vi "delete me.vi"() -> ()   [LabVIEW 2020]
uses:
  Shared/GUI_Template/GUI_master/tcp_new_data_event.ctl
  Shared/GUI_Template/GUI_master/tcp new data cluster.ctl
  <vilib>/Utility/file.llb/Read From Spreadsheet File (string).vi
panel:
  out "millisecond timer value":u32
  out "appended path":path
  in  "GUIdevice 98":string="PicoPad4"
  in  "Position.Axis 111::98":dbl=77.0 caption="Motor Axis 1" min=-30000.0 max=30000.0 format="%#_6f"
  in  "Position.Axis 112::98":dbl=77.0 caption="Motor Axis 1" min=-20000.0 max=20000.0 format="%#_6f"
  in  "Position.Axis 113::98":dbl=77.0 caption="Motor Axis 1" min=-20000.0 max=20000.0 format="%#_6f"
  in  "Position.Axis 121::98":dbl=77.0 caption="Motor Axis 1" min=-999999.0 max=999999.0 format="%#_6f"
  in  "Position.Axis 122::98":dbl=77.0 caption="Motor Axis 1" min=-999999.0 max=999999.0 format="%#_6f"
  in  "Position.Axis 123::98":dbl=77.0 caption="Motor Axis 1" min=-999999.0 max=999999.0 format="%#_6f"
  in  "Position.Axis 131::98":dbl=77.0 caption="Motor Axis 1" min=-999999.0 max=999999.0 format="%#_6f"
  in  "Position.Axis 132::98":dbl=77.0 caption="Motor Axis 1" min=-999999.0 max=999999.0 format="%#_6f"
  in  "Position.Axis 133::98":dbl=77.0 caption="Motor Axis 1" min=-999999.0 max=999999.0 format="%#_6f"
  in  "Position.Axis 141::98":dbl=77.0 caption="Motor Axis 1" min=-999999.0 max=999999.0 format="%#_6f"
  in  "Position.Axis 142::98":dbl=77.0 caption="Motor Axis 1" min=-999999.0 max=999999.0 format="%#_6f"
  in  "Position.Axis 143::98":dbl=77.0 caption="Motor Axis 1" min=-999999.0 max=999999.0 format="%#_6f"
  in  "Position.Axis 211::98":dbl=77.0 caption="Motor Axis 1" min=-999999.0 max=999999.0 format="%#_6f"
  in  "Position.Axis 212::98":dbl=77.0 caption="Motor Axis 1" min=-999999.0 max=999999.0 format="%#_6f"
  in  "Position.Axis 213::98":dbl=77.0 caption="Motor Axis 1" min=-999999.0 max=999999.0 format="%#_6f"
  in  "Position.Axis 221::98":dbl=77.0 caption="Motor Axis 1" min=-999999.0 max=999999.0 format="%#_6f"
  in  "Position.Axis 222::98":dbl=77.0 caption="Motor Axis 1" min=-999999.0 max=999999.0 format="%#_6f"
  in  "Position.Axis 223::98":dbl=77.0 caption="Motor Axis 1" min=-999999.0 max=999999.0 format="%#_6f"
  in  "Position.Axis 231::98":dbl=77.0 caption="Motor Axis 1" min=-999999.0 max=999999.0 format="%#_6f"
  in  "Position.Axis 232::98":dbl=77.0 caption="Motor Axis 1" min=-999999.0 max=999999.0 format="%#_6f"
  in  "Position.Axis 233::98":dbl=77.0 caption="Motor Axis 1" min=-999999.0 max=999999.0 format="%#_6f"
  in  "Position.Axis 241::98":dbl=77.0 caption="Motor Axis 1" min=-999999.0 max=999999.0 format="%#_6f"
  in  "Position.Axis 242::98":dbl=77.0 caption="Motor Axis 1" min=-999999.0 max=999999.0 format="%#_6f"
  in  "Position.Axis 243::98":dbl=77.0 caption="Motor Axis 1" min=-999999.0 max=999999.0 format="%#_6f"
  in  "Position.Axis 311::98":dbl=77.0 caption="Motor Axis 1" min=-999999.0 max=999999.0 format="%#_6f"
  in  "Position.Axis 312::98":dbl=77.0 caption="Motor Axis 1" min=-999999.0 max=999999.0 format="%#_6f"
  in  "Position.Axis 313::98":dbl=77.0 caption="Motor Axis 1" min=-999999.0 max=999999.0 format="%#_6f"
  in  "Position.Axis 321::98":dbl=77.0 caption="Motor Axis 1" min=-999999.0 max=999999.0 format="%#_6f"
  in  "Position.Axis 322::98":dbl=77.0 caption="Motor Axis 1" min=-999999.0 max=999999.0 format="%#_6f"
  in  "Position.Axis 323::98":dbl=77.0 caption="Motor Axis 1" min=-999999.0 max=999999.0 format="%#_6f"
  in  "Position.Axis 331::98":dbl=77.0 caption="Motor Axis 1" min=-999999.0 max=999999.0 format="%#_6f"
  in  "Position.Axis 332::98":dbl=77.0 caption="Motor Axis 1" min=-999999.0 max=999999.0 format="%#_6f"
  in  "Position.Axis 333::98":dbl=77.0 caption="Motor Axis 1" min=-999999.0 max=999999.0 format="%#_6f"
  in  "Position.Axis 341::98":dbl=77.0 caption="Motor Axis 1" min=-999999.0 max=999999.0 format="%#_6f"
  in  "Position.Axis 342::98":dbl=77.0 caption="Motor Axis 1" min=-999999.0 max=999999.0 format="%#_6f"
  in  "Position.Axis 343::98":dbl=77.0 caption="Motor Axis 1" min=-999999.0 max=999999.0 format="%#_6f"
  in  "Position.Axis 411::98":dbl=77.0 caption="Motor Axis 1" min=-999999.0 max=999999.0 format="%#_6f"
  in  "Position.Axis 412::98":dbl=77.0 caption="Motor Axis 1" min=-999999.0 max=999999.0 format="%#_6f"
  in  "Position.Axis 413::98":dbl=77.0 caption="Motor Axis 1" min=-999999.0 max=999999.0 format="%#_6f"
  in  "Position.Axis 421::98":dbl=77.0 caption="Motor Axis 1" min=-999999.0 max=999999.0 format="%#_6f"
  in  "Position.Axis 422::98":dbl=77.0 caption="Motor Axis 1" min=-999999.0 max=999999.0 format="%#_6f"
  in  "Position.Axis 423::98":dbl=77.0 caption="Motor Axis 1" min=-999999.0 max=999999.0 format="%#_6f"
  in  "Position.Axis 431::98":dbl=77.0 caption="Motor Axis 1" min=-999999.0 max=999999.0 format="%#_6f"
  in  "Position.Axis 432::98":dbl=77.0 caption="Motor Axis 1" min=-999999.0 max=999999.0 format="%#_6f"
  in  "Position.Axis 433::98":dbl=77.0 caption="Motor Axis 1" min=-999999.0 max=999999.0 format="%#_6f"
  in  "Position.Axis 441::98":dbl=77.0 caption="Motor Axis 1" min=-999999.0 max=999999.0 format="%#_6f"
  in  "Position.Axis 442::98":dbl=77.0 caption="Motor Axis 1" min=-999999.0 max=999999.0 format="%#_6f"
  in  "Position.Axis 443::98":dbl=77.0 caption="Motor Axis 1" min=-999999.0 max=999999.0 format="%#_6f"
  in  "Position.Axis 511::98":dbl=77.0 caption="Motor Axis 1" min=-999999.0 max=999999.0 format="%#_6f"
  in  "Position.Axis 512::98":dbl=77.0 caption="Motor Axis 1" min=-999999.0 max=999999.0 format="%#_6f"
  in  "Position.Axis 513::98":dbl=77.0 caption="Motor Axis 1" min=-999999.0 max=999999.0 format="%#_6f"
  in  "Position.Axis 521::98":dbl=77.0 caption="Motor Axis 1" min=-999999.0 max=999999.0 format="%#_6f"
  in  "Position.Axis 522::98":dbl=77.0 caption="Motor Axis 1" min=-999999.0 max=999999.0 format="%#_6f"
  in  "Position.Axis 523::98":dbl=77.0 caption="Motor Axis 1" min=-999999.0 max=999999.0 format="%#_6f"
  in  "Position.Axis 531::98":dbl=77.0 caption="Motor Axis 1" min=-999999.0 max=999999.0 format="%#_6f"
  in  "Position.Axis 532::98":dbl=77.0 caption="Motor Axis 1" min=-999999.0 max=999999.0 format="%#_6f"
  in  "Position.Axis 533::98":dbl=77.0 caption="Motor Axis 1" min=-999999.0 max=999999.0 format="%#_6f"
  in  "Position.Axis 541::98":dbl=77.0 caption="Motor Axis 1" min=-999999.0 max=999999.0 format="%#_6f"
  in  "Position.Axis 542::98":dbl=77.0 caption="Motor Axis 1" min=-999999.0 max=999999.0 format="%#_6f"
  in  "Position.Axis 543::98":dbl=77.0 caption="Motor Axis 1" min=-999999.0 max=999999.0 format="%#_6f"
  in  "Numeric":dbl
  out "CCDs":string[](array[string])
  in  "GUIdevice 12":string
  in  "GUIdevice 11":string
  in  "GUIdevice 10":string
  in  "GUIdevice 9":string
  out "error out 2":errorcluster
  out "Names":string[](array[string])
  in  "Tab Control 2":enum32{"Config ", "Main", "History"}(tab)=enum."Main"
  out "Cameras":T1
  in  "Exposure:12":dbl=0.095 min=0.0001 max=1.0 format="%#_6f"
  in  "Triggerdelay::12":dbl=0.003 min=0.0 max=0.09 format="%#_6f"
  in  "Exposure::11":dbl=0.095 min=0.0001 max=1.0 format="%#_6f"
  in  "Triggerdelay::11":dbl=0.003 min=0.0 max=0.09 format="%#_6f"
  in  "Exposure::10":dbl=0.095 min=0.0001 max=1.0 format="%#_6f"
  in  "Triggerdelay::10":dbl=0.003 min=0.0 max=0.09 format="%#_6f"
  in  "Exposure::9":dbl=0.095 min=0.0001 max=1.0 format="%#_6f"
  in  "Triggerdelay::9":dbl=0.003 min=0.0 max=0.09 format="%#_6f"
  in  "Trigger::9":bool
  in  "Trigger::10":bool caption="Trigger:10"
  in  "Trigger::11":bool
  in  "Trigger::12":bool
  in  "Exposure::8":dbl=0.095 caption="sdgdfg" min=0.0001 max=1.0 format="%#_6f"
  in  "Triggerdelay::8":dbl=0.003 caption="sdfsd" min=0.0 max=0.09 format="%#_6f"
  in  "Trigger::8":bool
  in  "Exposure::7":dbl=0.095 caption="dfgdf" min=0.0001 max=1.0 format="%#_6f"
  in  "Triggerdelay::7":dbl=0.003 caption="dfgdfg" min=0.0 max=0.09 format="%#_6f"
  in  "Trigger::7":bool
  in  "Exposure::6":dbl=0.095 caption="dfgdfg" min=0.0001 max=1.0 format="%#_6f"
  in  "Triggerdelay::6":dbl=0.003 caption="dfgdfg" min=0.0 max=0.09 format="%#_6f"
  in  "Trigger::6":bool
  in  "Exposure::5":dbl=0.095 caption="dfgfd" min=1e-05 max=2.0 format="%#_6f"
  in  "Triggerdelay::5":dbl=0.003 caption="dfgdf" min=0.0 max=100000.0 format="%#_6f"
  in  "Trigger::5":bool
  in  "Exposure::4":dbl=0.095 caption="dfgdf" min=0.0001 max=1.0 format="%#_6f"
  in  "Triggerdelay::4":dbl=0.003 caption="dfgdfgfd" min=0.0 max=0.09 format="%#_6f"
  in  "Trigger::4":bool
  in  "Exposure::3":dbl=0.095 caption="dfgdf" min=1e-05 max=2.0 format="%#_6f"
  in  "Triggerdelay::3":dbl=0.003 caption="dfgdfg" min=0.0 max=0.09 format="%#_6f"
  in  "Trigger::3":bool
  in  "Exposure::2":dbl=0.095 caption="gfdg" min=0.0001 max=1.0 format="%#_6f"
  in  "Triggerdelay::2":dbl=0.003 caption="dfgdfg" min=0.0 max=0.09 format="%#_6f"
  in  "Trigger::2":bool
  out "image::1":T2(plugin-control) caption="regen-out-cam"
  out "image::2":T2(plugin-control) caption="xpw-cam"
  out "image::3":T2(plugin-control) caption="xpw-out-cam"
  out "image::4":T2(plugin-control) caption="amp0-out-cam"
  out "image::5":T2(plugin-control) caption="preamp-in-cam"
  out "image::6":T2(plugin-control) caption="preamp-2nd-pass-cam"
  out "image::7":T2(plugin-control) caption="compressor-in-cam"
  out "image::8":T2(plugin-control) caption="compressor-out-cam"
  in  "Exposure::1":dbl=0.095 caption="exposure" min=0.0001 max=1.0 format="%#_6f"
  in  "Triggerdelay::1":dbl=0.003 caption="trig delay" min=0.0 max=0.09 format="%#_6f"
  in  "Trigger::1":bool
  in  "UDP error message":string
  out "image::9":T2(plugin-control)
  out "image::10":T2(plugin-control)
  out "image::11":T2(plugin-control)
  out "image::12":T2(plugin-control)
  in  "Feedback Global":bool
  in  "GUIdevice 8":string="B5_CompressorOut"
  in  "Tab Control":T3(tab)
  in  "Center":bool
  in  "Save Stats":bool
  in  "Save Config":bool
  in  "Load Config":bool
  in  "Img to avg":i32=3 min=3 max=200
  in  "Reset History":bool
  in  "new tdms":bool
  in  "deivice ini":bool
  in  "RelativeMove.Axis 1.CCW::99":bool caption="RelativeMove.Axis 1.CCW::1"
  in  "RelativeMove.Axis 1.CW::99":bool caption="RelativeMove.Axis 1.CW::1"
  in  "RelativeMove.Axis 2.CCW::99":bool caption="RelativeMove.Axis. 2.CCW::1"
  in  "RelativeMove.Axis 2.CW::99":bool caption="RelativeMove.Axis 2.CW::1"
  in  "RelativeSettings.Axis 1.Position::99":dbl caption="Axis 1 Position" min=-999999.0 max=999999.0 format="%_4p"
  in  "RelativeSettings.Axis 2.Position::99":dbl caption="Axis 2 Position" min=-999999.0 max=999999.0 format="%_4p"
  in  "RelativeSettings.Axis 2.StepSize::99":dbl=50.0 caption="Axis 2 StepSize" min=0.0 max=999999.0 format="%_4p"
  in  "RelativeSettings.Axis 1.StepSize::99":dbl=50.0 caption="Axis 1 Stepsize" min=0.0 max=999999.0 format="%_4p"
  in  "CCDs":u16(ring) items=["regen-out-cam", "xpw-cam", "xpw-out-cam", "amp0-out-cam", "preamp-in-cam", "preamp-2nd-pass-cam", "compressor-in-cam", "compressor-out-cam", "", "", "", ""]
  out "motor refs":refnum<vi>[](array[refnum])
  in  "Position.Axis 511::99":dbl=77.0 caption="Motor Axis 1" min=-999999.0 max=999999.0 format="%#_6f"
  in  "Position.Axis 512::99":dbl=77.0 caption="Motor Axis 1" min=-999999.0 max=999999.0 format="%#_6f"
  in  "Position.Axis 513::99":dbl=77.0 caption="Motor Axis 1" min=-999999.0 max=999999.0 format="%#_6f"
  in  "Position.Axis 521::99":dbl=77.0 caption="Motor Axis 1" min=-999999.0 max=999999.0 format="%#_6f"
  in  "Position.Axis 522::99":dbl=77.0 caption="Motor Axis 1" min=-999999.0 max=999999.0 format="%#_6f"
  in  "Position.Axis 523::99":dbl=77.0 caption="Motor Axis 1" min=-999999.0 max=999999.0 format="%#_6f"
  in  "Position.Axis 531::99":dbl=77.0 caption="Motor Axis 1" min=-999999.0 max=999999.0 format="%#_6f"
  in  "Position.Axis 532::99":dbl=77.0 caption="Motor Axis 1" min=-999999.0 max=999999.0 format="%#_6f"
  in  "Position.Axis 533::99":dbl=77.0 caption="Motor Axis 1" min=-999999.0 max=999999.0 format="%#_6f"
  in  "Position.Axis 541::99":dbl=77.0 caption="Motor Axis 1" min=-999999.0 max=999999.0 format="%#_6f"
  in  "Position.Axis 542::99":dbl=77.0 caption="Motor Axis 1" min=-999999.0 max=999999.0 format="%#_6f"
  in  "Position.Axis 543::99":dbl=77.0 caption="Motor Axis 1" min=-999999.0 max=999999.0 format="%#_6f"
  in  "Position.Axis 411::99":dbl=77.0 caption="Motor Axis 1" min=-999999.0 max=999999.0 format="%#_6f"
  in  "Position.Axis 412::99":dbl=77.0 caption="Motor Axis 1" min=-999999.0 max=999999.0 format="%#_6f"
  in  "Position.Axis 413::99":dbl=77.0 caption="Motor Axis 1" min=-999999.0 max=999999.0 format="%#_6f"
  in  "Position.Axis 421::99":dbl=77.0 caption="Motor Axis 1" min=-999999.0 max=999999.0 format="%#_6f"
  in  "Position.Axis 422::99":dbl=77.0 caption="Motor Axis 1" min=-999999.0 max=999999.0 format="%#_6f"
  in  "Position.Axis 423::99":dbl=77.0 caption="Motor Axis 1" min=-999999.0 max=999999.0 format="%#_6f"
  in  "Position.Axis 431::99":dbl=77.0 caption="Motor Axis 1" min=-999999.0 max=999999.0 format="%#_6f"
  in  "Position.Axis 432::99":dbl=77.0 caption="Motor Axis 1" min=-999999.0 max=999999.0 format="%#_6f"
  in  "Position.Axis 433::99":dbl=77.0 caption="Motor Axis 1" min=-999999.0 max=999999.0 format="%#_6f"
  in  "Position.Axis 441::99":dbl=77.0 caption="Motor Axis 1" min=-999999.0 max=999999.0 format="%#_6f"
  in  "Position.Axis 442::99":dbl=77.0 caption="Motor Axis 1" min=-999999.0 max=999999.0 format="%#_6f"
  in  "Position.Axis 443::99":dbl=77.0 caption="Motor Axis 1" min=-999999.0 max=999999.0 format="%#_6f"
  in  "Position.Axis 311::99":dbl=77.0 caption="Motor Axis 1" min=-999999.0 max=999999.0 format="%#_6f"
  in  "Position.Axis 312::99":dbl=77.0 caption="Motor Axis 1" min=-999999.0 max=999999.0 format="%#_6f"
  in  "Position.Axis 313::99":dbl=77.0 caption="Motor Axis 1" min=-999999.0 max=999999.0 format="%#_6f"
  in  "Position.Axis 321::99":dbl=77.0 caption="Motor Axis 1" min=-999999.0 max=999999.0 format="%#_6f"
  in  "Position.Axis 322::99":dbl=77.0 caption="Motor Axis 1" min=-999999.0 max=999999.0 format="%#_6f"
  in  "Position.Axis 323::99":dbl=77.0 caption="Motor Axis 1" min=-999999.0 max=999999.0 format="%#_6f"
  in  "Position.Axis 331::99":dbl=77.0 caption="Motor Axis 1" min=-999999.0 max=999999.0 format="%#_6f"
  in  "Position.Axis 332::99":dbl=77.0 caption="Motor Axis 1" min=-999999.0 max=999999.0 format="%#_6f"
  in  "Position.Axis 333::99":dbl=77.0 caption="Motor Axis 1" min=-999999.0 max=999999.0 format="%#_6f"
  in  "Position.Axis 341::99":dbl=77.0 caption="Motor Axis 1" min=-999999.0 max=999999.0 format="%#_6f"
  in  "Position.Axis 342::99":dbl=77.0 caption="Motor Axis 1" min=-999999.0 max=999999.0 format="%#_6f"
  in  "Position.Axis 343::99":dbl=77.0 caption="Motor Axis 1" min=-999999.0 max=999999.0 format="%#_6f"
  in  "Position.Axis 241::99":dbl=77.0 caption="Motor Axis 1" min=-999999.0 max=999999.0 format="%#_6f"
  in  "Position.Axis 242::99":dbl=77.0 caption="Motor Axis 1" min=-999999.0 max=999999.0 format="%#_6f"
  in  "Position.Axis 243::99":dbl=77.0 caption="Motor Axis 1" min=-999999.0 max=999999.0 format="%#_6f"
  in  "Position.Axis 231::99":dbl=77.0 caption="Motor Axis 1" min=-999999.0 max=999999.0 format="%#_6f"
  in  "Position.Axis 232::99":dbl=77.0 caption="Motor Axis 1" min=-999999.0 max=999999.0 format="%#_6f"
  in  "Position.Axis 233::99":dbl=77.0 caption="Motor Axis 1" min=-999999.0 max=999999.0 format="%#_6f"
  in  "Position.Axis 221::99":dbl=77.0 caption="Motor Axis 1" min=-999999.0 max=999999.0 format="%#_6f"
  in  "Position.Axis 222::99":dbl=77.0 caption="Motor Axis 1" min=-999999.0 max=999999.0 format="%#_6f"
  in  "Position.Axis 223::99":dbl=77.0 caption="Motor Axis 1" min=-999999.0 max=999999.0 format="%#_6f"
  in  "Position.Axis 211::99":dbl=77.0 caption="Motor Axis 1" min=-999999.0 max=999999.0 format="%#_6f"
  in  "Position.Axis 212::99":dbl=77.0 caption="Motor Axis 1" min=-999999.0 max=999999.0 format="%#_6f"
  in  "Position.Axis 213::99":dbl=77.0 caption="Motor Axis 1" min=-999999.0 max=999999.0 format="%#_6f"
  in  "Position.Axis 141::99":dbl=77.0 caption="Motor Axis 1" min=-999999.0 max=999999.0 format="%#_6f"
  in  "Position.Axis 142::99":dbl=77.0 caption="Motor Axis 1" min=-999999.0 max=999999.0 format="%#_6f"
  in  "Position.Axis 143::99":dbl=77.0 caption="Motor Axis 1" min=-999999.0 max=999999.0 format="%#_6f"
  in  "Position.Axis 131::99":dbl=77.0 caption="Motor Axis 1" min=-999999.0 max=999999.0 format="%#_6f"
  in  "Position.Axis 132::99":dbl=77.0 caption="Motor Axis 1" min=-999999.0 max=999999.0 format="%#_6f"
  in  "Position.Axis 133::99":dbl=77.0 caption="Motor Axis 1" min=-999999.0 max=999999.0 format="%#_6f"
  in  "Position.Axis 121::99":dbl=77.0 caption="Motor Axis 1" min=-999999.0 max=999999.0 format="%#_6f"
  in  "Position.Axis 122::99":dbl=77.0 caption="Motor Axis 1" min=-999999.0 max=999999.0 format="%#_6f"
  in  "Position.Axis 123::99":dbl=77.0 caption="Motor Axis 1" min=-999999.0 max=999999.0 format="%#_6f"
  in  "Position.Axis 113::99":dbl=77.0 caption="Motor Axis 1" min=-999999.0 max=999999.0 format="%#_6f"
  in  "Position.Axis 112::99":dbl=77.0 caption="Motor Axis 1" min=-999999.0 max=999999.0 format="%#_6f"
  in  "Position.Axis 111::99":dbl=77.0 caption="Motor Axis 1" min=-999999.0 max=999999.0 format="%#_6f"
  in  "GUIdevice 99":string="Picopad23"
  in  "active CCDs":i32(listbox)=1
  in  "GUIdevice 7":string="B2_TelLens1"
  in  "GUIdevice 6":string="B1_TelInput"
  in  "GUIdevice 5":string="L8_M10Leak"
  in  "GUIdevice 4":string="L7_TREXPass4"
  in  "GUIdevice 3":string="L6_TREXpass3"
  in  "GUIdevice 2":string="L5_TREXPass2"
  in  "insert tag":bool=TRUE
  in  "stop":bool
  in  "GUIdevice 1":string="L4_TREXpass1"
  out "tcp data event":T4
  out "error IO 2":errorcluster
  # "x [Tolerance]"
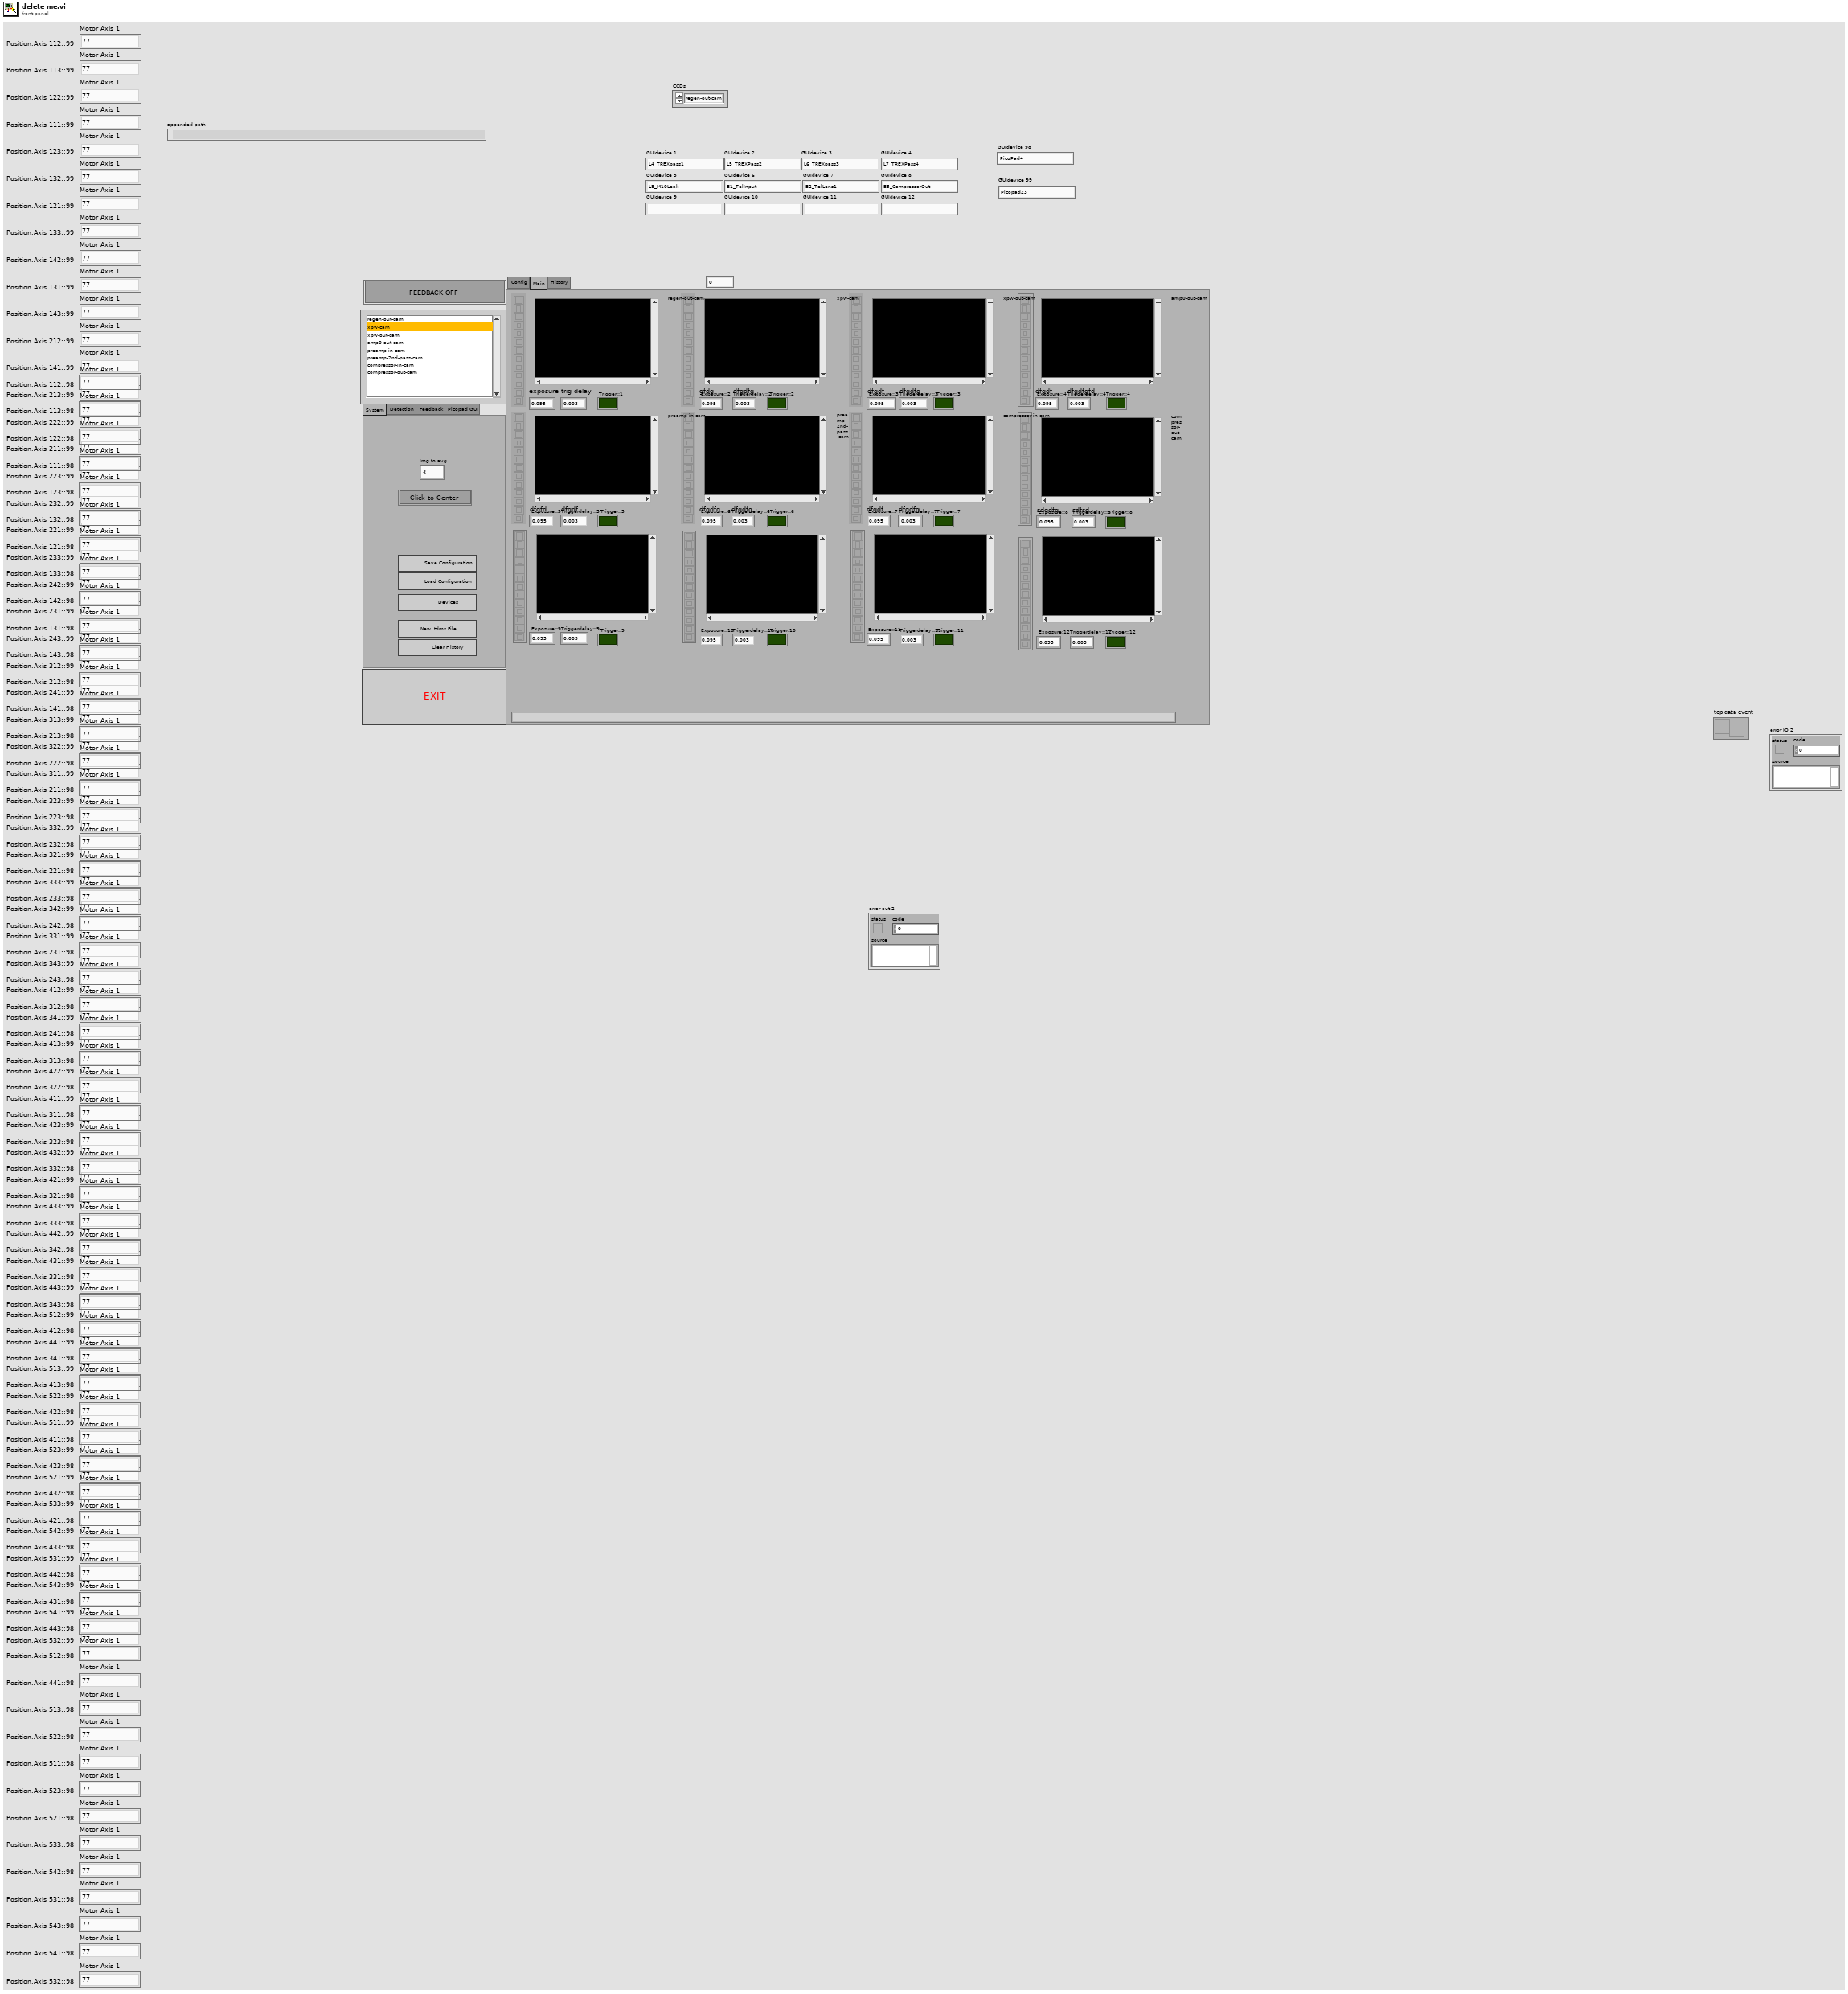
[diagram p1: front panel]
types:
  T1 = cluster{"[0]":string, "[1]":string, "[2]":string, "[3]":string, "[4]":string, "[5]":string, "[6]":string, "[7]":string, "[8]":string, "[8] 2":string, "[8] 3":string, "[8] 4":string}
  T2 = typedef "IMAQ Image.ctl" = refnum<image>
  T3 = enum32{"System", "Detection", "Feedback", "Picopad GUI"}
  T4 = typedef "tcp_new_data_event.ctl" = refnum<user-event>
  T5 = typedef "tcp new data cluster.ctl" = cluster{"EventEnum":enum16{"new data", "connection status update"}, "Device name":string}
  T6 = typedef "Image Type" = u32
  T7 = cluster{"[0]":string, "[1]":string, "[2]":string, "[3]":string, "[4]":string, "[5]":string, "[6]":string, "[7]":string, "[8]":string, "[9]":string, "[10]":string, "[11]":string}
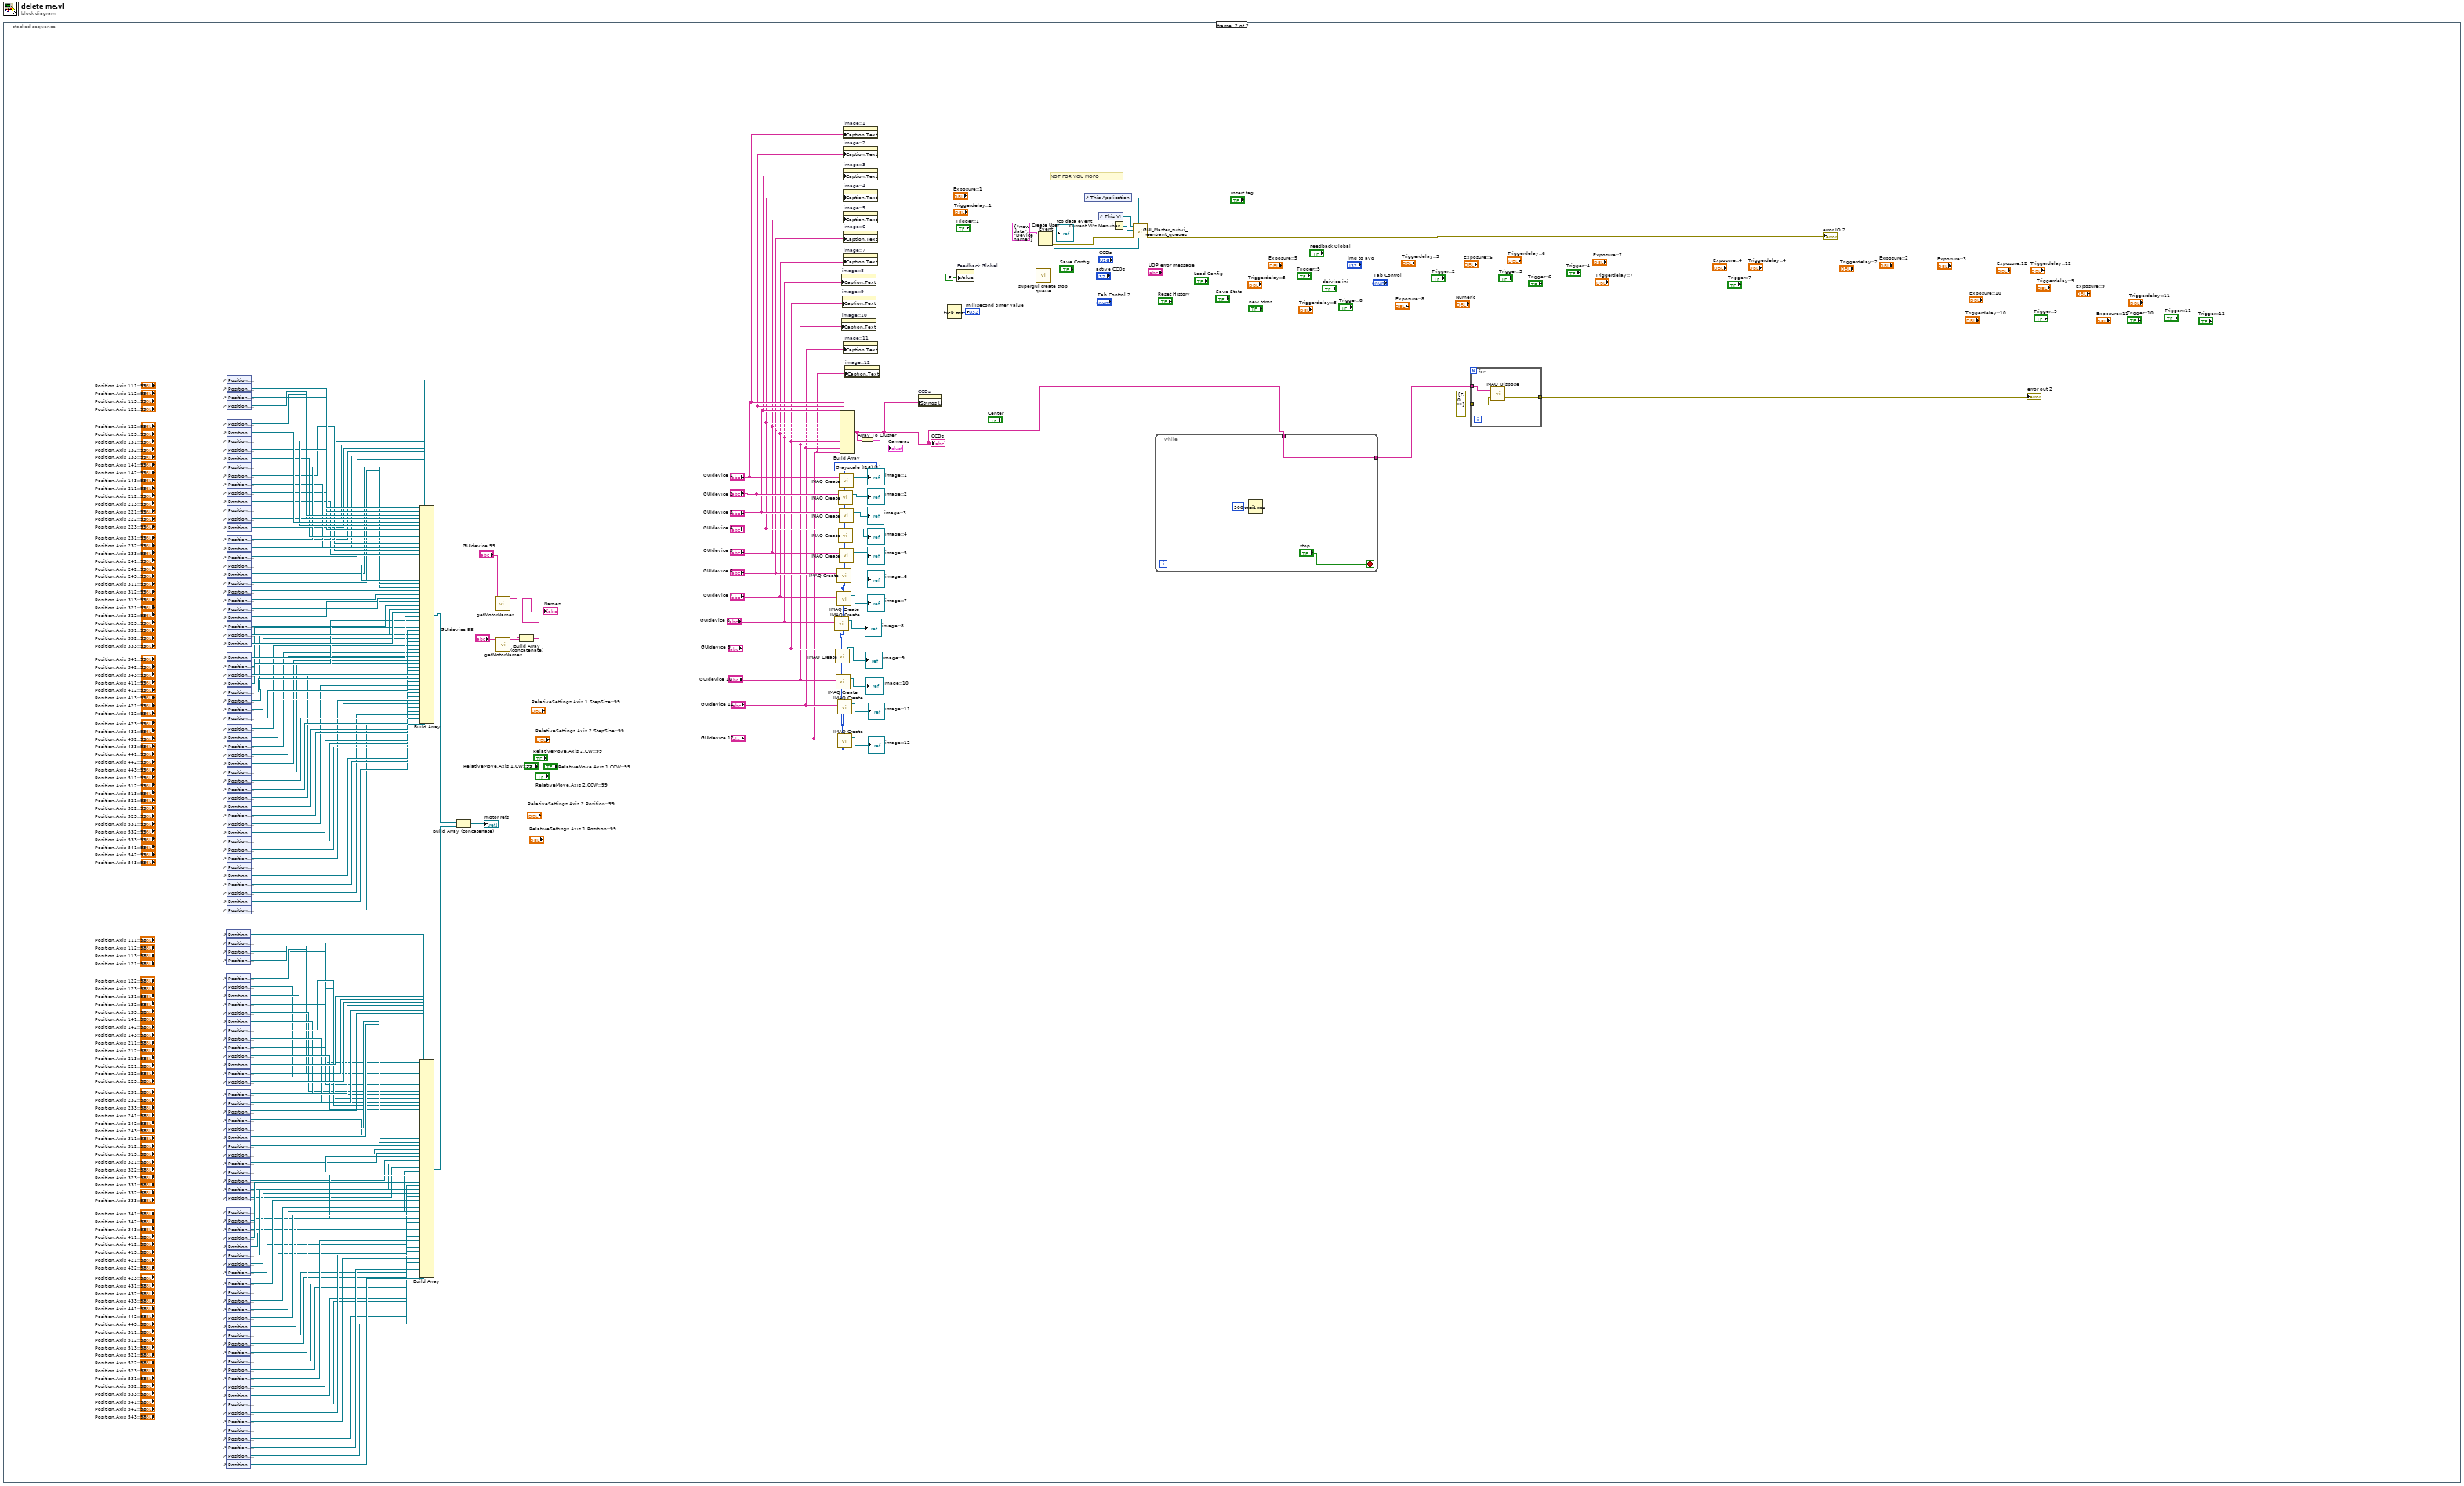
[diagram p0: block diagram]
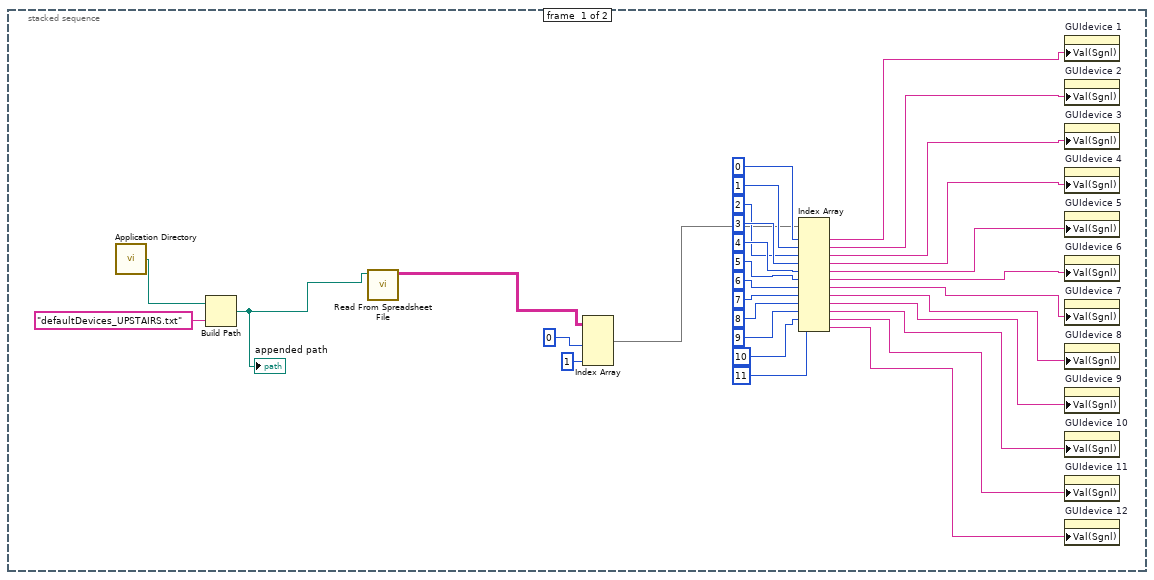
[diagram p2: hidden frame]
diagram:
  n1 = stacked-sequence {
    frame #0 {
      n2 = call <vilib>:"Application Directory.vi"() -> ("Application Directory"=w13:path)
      n3 = Build Path(base path=w13, name or relative path="defaultDevices_UPSTAIRS.txt") -> (appended path=w15:path)
      "appended path" <- w15
      n4 = call-poly <vilib>:"Read From Spreadsheet File.vi"("file path (dialog if empty)"=w15) -> ("all rows"=w16:string[][])  [unwired: 6 in, 4 out]
      n5 = Index Array(array=w16, index (col) #1=0 ("disabled index (col)"), index (col) #2=1 ("index (col)")) -> (element #1=w19:string[])  [unwired: 2 in, 1 out]
      n6 = Index Array(array=w19, index #1=0 ("index"), index #2=1 ("index"), index #3=2 ("index"), index #4=3 ("index"), index #5=4 ("index"), index #6=5 ("index"), index #7=6 ("index"), index #8=7 ("index"), index #9=8 ("index"), index #10=9 ("index"), index #11=10 ("index"), index #12=11 ("index")) -> (element #1=w12:string, element #2=w11:string, element #3=w10:string, element #4=w9:string, element #5=w8:string, element #6=w7:string, element #7=w6:string, element #8=w5:string, element #9=w4:string, element #10=w3:string, element #11=w2:string, element #12=w1:string)
      n7 = property on="GUIdevice 1" class="Str"("Val(Sgnl)"=w12) -> ()  [unwired: 2 in, 2 out]
      n8 = property on="GUIdevice 2" class="Str"("Val(Sgnl)"=w11) -> ()  [unwired: 2 in, 2 out]
      n9 = property on="GUIdevice 3" class="Str"("Val(Sgnl)"=w10) -> ()  [unwired: 2 in, 2 out]
      n10 = property on="GUIdevice 4" class="Str"("Val(Sgnl)"=w9) -> ()  [unwired: 2 in, 2 out]
      n11 = property on="GUIdevice 5" class="Str"("Val(Sgnl)"=w8) -> ()  [unwired: 2 in, 2 out]
      n12 = property on="GUIdevice 6" class="Str"("Val(Sgnl)"=w7) -> ()  [unwired: 2 in, 2 out]
      n13 = property on="GUIdevice 7" class="Str"("Val(Sgnl)"=w6) -> ()  [unwired: 2 in, 2 out]
      n14 = property on="GUIdevice 8" class="Str"("Val(Sgnl)"=w5) -> ()  [unwired: 2 in, 2 out]
      n15 = property on="GUIdevice 9" class="Str"("Val(Sgnl)"=w4) -> ()  [unwired: 2 in, 2 out]
      n16 = property on="GUIdevice 10" class="Str"("Val(Sgnl)"=w3) -> ()  [unwired: 2 in, 2 out]
      n17 = property on="GUIdevice 11" class="Str"("Val(Sgnl)"=w2) -> ()  [unwired: 2 in, 2 out]
      n18 = property on="GUIdevice 12" class="Str"("Val(Sgnl)"=w1) -> ()  [unwired: 2 in, 2 out]
    }
    frame #1 {
      w107 = T6 1 items=["Grayscale (U8)", "Grayscale (I16)", "Grayscale (SGL)", "Complex (CSG)", "RGB (U32)", "HSL (U32)", "RGB (U64)", "Grayscale (U16)"] ("Image Type")
      # "NOT FOR YOU MOFO"
      n19 = control-ref of="Position.Axis 111::98"() -> (w44:refnum<vi>)
      n20 = control-ref of="Position.Axis 112::98"() -> (w45:refnum<vi>)
      n21 = control-ref of="Position.Axis 113::98"() -> (w46:refnum<vi>)
      n22 = control-ref of="Position.Axis 121::98"() -> (w47:refnum<vi>)
      n23 = control-ref of="Position.Axis 122::98"() -> (w48:refnum<vi>)
      n24 = control-ref of="Position.Axis 123::98"() -> (w49:refnum<vi>)
      n25 = control-ref of="Position.Axis 131::98"() -> (w50:refnum<vi>)
      n26 = control-ref of="Position.Axis 132::98"() -> (w51:refnum<vi>)
      n27 = control-ref of="Position.Axis 133::98"() -> (w52:refnum<vi>)
      n28 = control-ref of="Position.Axis 141::98"() -> (w53:refnum<vi>)
      n29 = control-ref of="Position.Axis 142::98"() -> (w54:refnum<vi>)
      n30 = control-ref of="Position.Axis 143::98"() -> (w55:refnum<vi>)
      n31 = control-ref of="Position.Axis 211::98"() -> (w56:refnum<vi>)
      n32 = control-ref of="Position.Axis 212::98"() -> (w57:refnum<vi>)
      n33 = control-ref of="Position.Axis 213::98"() -> (w58:refnum<vi>)
      n34 = control-ref of="Position.Axis 221::98"() -> (w59:refnum<vi>)
      n35 = control-ref of="Position.Axis 222::98"() -> (w60:refnum<vi>)
      n36 = control-ref of="Position.Axis 223::98"() -> (w61:refnum<vi>)
      n37 = control-ref of="Position.Axis 231::98"() -> (w62:refnum<vi>)
      n38 = control-ref of="Position.Axis 232::98"() -> (w63:refnum<vi>)
      n39 = control-ref of="Position.Axis 233::98"() -> (w64:refnum<vi>)
      n40 = control-ref of="Position.Axis 241::98"() -> (w65:refnum<vi>)
      n41 = control-ref of="Position.Axis 242::98"() -> (w66:refnum<vi>)
      n42 = control-ref of="Position.Axis 243::98"() -> (w67:refnum<vi>)
      n43 = control-ref of="Position.Axis 311::98"() -> (w68:refnum<vi>)
      n44 = control-ref of="Position.Axis 312::98"() -> (w69:refnum<vi>)
      n45 = control-ref of="Position.Axis 313::98"() -> (w70:refnum<vi>)
      n46 = control-ref of="Position.Axis 321::98"() -> (w71:refnum<vi>)
      n47 = control-ref of="Position.Axis 322::98"() -> (w72:refnum<vi>)
      n48 = control-ref of="Position.Axis 323::98"() -> (w73:refnum<vi>)
      n49 = control-ref of="Position.Axis 331::98"() -> (w74:refnum<vi>)
      n50 = control-ref of="Position.Axis 332::98"() -> (w75:refnum<vi>)
      n51 = control-ref of="Position.Axis 333::98"() -> (w76:refnum<vi>)
      n52 = control-ref of="Position.Axis 341::98"() -> (w77:refnum<vi>)
      n53 = control-ref of="Position.Axis 342::98"() -> (w78:refnum<vi>)
      n54 = control-ref of="Position.Axis 343::98"() -> (w79:refnum<vi>)
      n55 = control-ref of="Position.Axis 411::98"() -> (w80:refnum<vi>)
      n56 = control-ref of="Position.Axis 412::98"() -> (w81:refnum<vi>)
      n57 = control-ref of="Position.Axis 413::98"() -> (w82:refnum<vi>)
      n58 = control-ref of="Position.Axis 421::98"() -> (w83:refnum<vi>)
      n59 = control-ref of="Position.Axis 422::98"() -> (w84:refnum<vi>)
      n60 = control-ref of="Position.Axis 423::98"() -> (w85:refnum<vi>)
      n61 = control-ref of="Position.Axis 431::98"() -> (w86:refnum<vi>)
      n62 = control-ref of="Position.Axis 432::98"() -> (w87:refnum<vi>)
      n63 = control-ref of="Position.Axis 433::98"() -> (w88:refnum<vi>)
      n64 = control-ref of="Position.Axis 441::98"() -> (w89:refnum<vi>)
      n65 = control-ref of="Position.Axis 442::98"() -> (w90:refnum<vi>)
      n66 = control-ref of="Position.Axis 443::98"() -> (w91:refnum<vi>)
      n67 = control-ref of="Position.Axis 511::98"() -> (w92:refnum<vi>)
      n68 = control-ref of="Position.Axis 512::98"() -> (w93:refnum<vi>)
      n69 = control-ref of="Position.Axis 513::98"() -> (w94:refnum<vi>)
      n70 = control-ref of="Position.Axis 521::98"() -> (w95:refnum<vi>)
      n71 = control-ref of="Position.Axis 522::98"() -> (w96:refnum<vi>)
      n72 = control-ref of="Position.Axis 523::98"() -> (w97:refnum<vi>)
      n73 = control-ref of="Position.Axis 531::98"() -> (w98:refnum<vi>)
      n74 = control-ref of="Position.Axis 532::98"() -> (w99:refnum<vi>)
      n75 = control-ref of="Position.Axis 533::98"() -> (w100:refnum<vi>)
      n76 = control-ref of="Position.Axis 541::98"() -> (w101:refnum<vi>)
      n77 = control-ref of="Position.Axis 542::98"() -> (w102:refnum<vi>)
      n78 = control-ref of="Position.Axis 543::98"() -> (w103:refnum<vi>)
      n79 = control-ref of="Position.Axis 111::99"() -> (w185:refnum<vi>)
      n80 = control-ref of="Position.Axis 112::99"() -> (w184:refnum<vi>)
      n81 = control-ref of="Position.Axis 113::99"() -> (w183:refnum<vi>)
      n82 = control-ref of="Position.Axis 121::99"() -> (w182:refnum<vi>)
      n83 = control-ref of="Position.Axis 122::99"() -> (w181:refnum<vi>)
      n84 = control-ref of="Position.Axis 123::99"() -> (w180:refnum<vi>)
      n85 = control-ref of="Position.Axis 131::99"() -> (w179:refnum<vi>)
      n86 = control-ref of="Position.Axis 132::99"() -> (w178:refnum<vi>)
      n87 = control-ref of="Position.Axis 133::99"() -> (w177:refnum<vi>)
      n88 = control-ref of="Position.Axis 141::99"() -> (w176:refnum<vi>)
      n89 = control-ref of="Position.Axis 142::99"() -> (w175:refnum<vi>)
      n90 = control-ref of="Position.Axis 143::99"() -> (w174:refnum<vi>)
      n91 = control-ref of="Position.Axis 211::99"() -> (w173:refnum<vi>)
      n92 = control-ref of="Position.Axis 212::99"() -> (w172:refnum<vi>)
      n93 = control-ref of="Position.Axis 213::99"() -> (w171:refnum<vi>)
      n94 = control-ref of="Position.Axis 221::99"() -> (w170:refnum<vi>)
      n95 = control-ref of="Position.Axis 222::99"() -> (w169:refnum<vi>)
      n96 = control-ref of="Position.Axis 223::99"() -> (w168:refnum<vi>)
      n97 = control-ref of="Position.Axis 231::99"() -> (w167:refnum<vi>)
      n98 = control-ref of="Position.Axis 232::99"() -> (w166:refnum<vi>)
      n99 = control-ref of="Position.Axis 233::99"() -> (w165:refnum<vi>)
      n100 = control-ref of="Position.Axis 241::99"() -> (w164:refnum<vi>)
      n101 = control-ref of="Position.Axis 242::99"() -> (w163:refnum<vi>)
      n102 = control-ref of="Position.Axis 243::99"() -> (w162:refnum<vi>)
      n103 = control-ref of="Position.Axis 311::99"() -> (w161:refnum<vi>)
      n104 = control-ref of="Position.Axis 312::99"() -> (w160:refnum<vi>)
      n105 = control-ref of="Position.Axis 313::99"() -> (w159:refnum<vi>)
      n106 = control-ref of="Position.Axis 321::99"() -> (w158:refnum<vi>)
      n107 = control-ref of="Position.Axis 322::99"() -> (w157:refnum<vi>)
      n108 = control-ref of="Position.Axis 323::99"() -> (w156:refnum<vi>)
      n109 = control-ref of="Position.Axis 331::99"() -> (w155:refnum<vi>)
      n110 = control-ref of="Position.Axis 332::99"() -> (w154:refnum<vi>)
      n111 = control-ref of="Position.Axis 333::99"() -> (w153:refnum<vi>)
      n112 = control-ref of="Position.Axis 341::99"() -> (w152:refnum<vi>)
      n113 = control-ref of="Position.Axis 342::99"() -> (w151:refnum<vi>)
      n114 = control-ref of="Position.Axis 343::99"() -> (w150:refnum<vi>)
      n115 = control-ref of="Position.Axis 411::99"() -> (w149:refnum<vi>)
      n116 = control-ref of="Position.Axis 412::99"() -> (w148:refnum<vi>)
      n117 = control-ref of="Position.Axis 413::99"() -> (w147:refnum<vi>)
      n118 = control-ref of="Position.Axis 421::99"() -> (w146:refnum<vi>)
      n119 = control-ref of="Position.Axis 422::99"() -> (w145:refnum<vi>)
      n120 = control-ref of="Position.Axis 423::99"() -> (w144:refnum<vi>)
      n121 = control-ref of="Position.Axis 431::99"() -> (w143:refnum<vi>)
      n122 = control-ref of="Position.Axis 432::99"() -> (w142:refnum<vi>)
      n123 = control-ref of="Position.Axis 433::99"() -> (w141:refnum<vi>)
      n124 = control-ref of="Position.Axis 441::99"() -> (w140:refnum<vi>)
      n125 = control-ref of="Position.Axis 442::99"() -> (w139:refnum<vi>)
      n126 = control-ref of="Position.Axis 443::99"() -> (w138:refnum<vi>)
      n127 = control-ref of="Position.Axis 511::99"() -> (w137:refnum<vi>)
      n128 = control-ref of="Position.Axis 512::99"() -> (w136:refnum<vi>)
      n129 = control-ref of="Position.Axis 513::99"() -> (w135:refnum<vi>)
      n130 = control-ref of="Position.Axis 521::99"() -> (w134:refnum<vi>)
      n131 = control-ref of="Position.Axis 522::99"() -> (w133:refnum<vi>)
      n132 = control-ref of="Position.Axis 523::99"() -> (w132:refnum<vi>)
      n133 = control-ref of="Position.Axis 531::99"() -> (w131:refnum<vi>)
      n134 = control-ref of="Position.Axis 532::99"() -> (w130:refnum<vi>)
      n135 = control-ref of="Position.Axis 533::99"() -> (w129:refnum<vi>)
      n136 = control-ref of="Position.Axis 541::99"() -> (w128:refnum<vi>)
      n137 = control-ref of="Position.Axis 542::99"() -> (w127:refnum<vi>)
      n138 = control-ref of="Position.Axis 543::99"() -> (w126:refnum<vi>)
      n139 = Build Array(w44, w45, w46, w47, w48, w49, w50, w51, w52, w53, w54, w55, w56, w57, w58, w59, w60, w61, w62, w63, w64, w65, w66, w67, w68, w69, w70, w71, w72, w73, w74, w75, w76, w77, w78, w79, w80, w81, w82, w83, w84, w85, w86, w87, w88, w89, w90, w91, w92, w93, w94, w95, w96, w97, w98, w99, w100, w101, w102, w103) -> (w41:refnum<vi>[])
      n140 = Build Array(w185, w184, w183, w182, w181, w180, w179, w178, w177, w176, w175, w174, w173, w172, w171, w170, w169, w168, w167, w166, w165, w164, w163, w162, w161, w160, w159, w158, w157, w156, w155, w154, w153, w152, w151, w150, w149, w148, w147, w146, w145, w144, w143, w142, w141, w140, w139, w138, w137, w136, w135, w134, w133, w132, w131, w130, w129, w128, w127, w126) -> (w40:refnum<vi>[])
      n141 = Build Array (concatenate)(w40, w41) -> (→"motor refs":refnum<vi>[])
      n142 = call "getMotorNames.vi"("DeviceName"="GUIdevice 99") -> ("elements"=w38:string[])  [unwired: 10 in]
      n143 = call "getMotorNames.vi"("DeviceName"="GUIdevice 98") -> ("elements"=w37:string[])  [unwired: 10 in]
      n144 = Build Array (concatenate)(w38, w37) -> (→"Names":string[])
      n145 = call "IMAQ Create"("Image Name"="GUIdevice 8", "Image Type"=w107) -> ("New Image"=→"image::8":T2)  [unwired: 3 in, 1 out]
      n146 = call "IMAQ Create"("Image Name"="GUIdevice 9", "Image Type"=w107) -> ("New Image"=→"image::9":T2)  [unwired: 3 in, 1 out]
      n147 = call "IMAQ Create"("Image Name"="GUIdevice 10", "Image Type"=w107) -> ("New Image"=→"image::10":T2)  [unwired: 3 in, 1 out]
      n148 = call "IMAQ Create"("Image Name"="GUIdevice 6", "Image Type"=w107) -> ("New Image"=→"image::6":T2)  [unwired: 3 in, 1 out]
      n149 = call "IMAQ Create"("Image Name"="GUIdevice 7", "Image Type"=w107) -> ("New Image"=→"image::7":T2)  [unwired: 3 in, 1 out]
      n150 = call "IMAQ Create"("Image Name"="GUIdevice 11", "Image Type"=w107) -> ("New Image"=→"image::11":T2)  [unwired: 3 in, 1 out]
      n151 = call "IMAQ Create"("Image Name"="GUIdevice 12", "Image Type"=w107) -> ("New Image"=→"image::12":T2)  [unwired: 3 in, 1 out]
      n152 = call "IMAQ Create"("Image Name"="GUIdevice 2") -> ("New Image"=→"image::2":T2)  [unwired: 4 in, 1 out]
      n153 = call "IMAQ Create"("Image Name"="GUIdevice 4", "Image Type"=w107) -> ("New Image"=→"image::4":T2)  [unwired: 3 in, 1 out]
      n154 = call "IMAQ Create"("Image Name"="GUIdevice 1", "Image Type"=w107) -> ("New Image"=→"image::1":T2)  [unwired: 3 in, 1 out]
      n155 = call "IMAQ Create"("Image Name"="GUIdevice 3", "Image Type"=w107) -> ("New Image"=→"image::3":T2)  [unwired: 3 in, 1 out]
      n156 = call "IMAQ Create"("Image Name"="GUIdevice 5", "Image Type"=w107) -> ("New Image"=→"image::5":T2)  [unwired: 3 in, 1 out]
      n157 = Build Array("GUIdevice 1", "GUIdevice 2", "GUIdevice 3", "GUIdevice 4", "GUIdevice 5", "GUIdevice 6", "GUIdevice 7", "GUIdevice 8", "GUIdevice 9", "GUIdevice 10", "GUIdevice 11", "GUIdevice 12") -> (w33:string[])
      "CCDs" <- w33
      n158 = property on="image::8" class="ImageControl"("Caption.Text"="GUIdevice 8") -> ()  [unwired: 2 in, 2 out]
      n159 = property on="image::10" class="ImageControl"("Caption.Text"="GUIdevice 10") -> ()  [unwired: 2 in, 2 out]
      n160 = property on="image::9" class="ImageControl"("Caption.Text"="GUIdevice 9") -> ()  [unwired: 2 in, 2 out]
      n161 = property on="image::1" class="ImageControl"("Caption.Text"="GUIdevice 1") -> ()  [unwired: 2 in, 2 out]
      n162 = property on="image::2" class="ImageControl"("Caption.Text"="GUIdevice 2") -> ()  [unwired: 2 in, 2 out]
      n163 = property on="image::3" class="ImageControl"("Caption.Text"="GUIdevice 3") -> ()  [unwired: 2 in, 2 out]
      n164 = property on="image::4" class="ImageControl"("Caption.Text"="GUIdevice 4") -> ()  [unwired: 2 in, 2 out]
      n165 = property on="image::5" class="ImageControl"("Caption.Text"="GUIdevice 5") -> ()  [unwired: 2 in, 2 out]
      n166 = property on="image::6" class="ImageControl"("Caption.Text"="GUIdevice 6") -> ()  [unwired: 2 in, 2 out]
      n167 = property on="image::7" class="ImageControl"("Caption.Text"="GUIdevice 7") -> ()  [unwired: 2 in, 2 out]
      n168 = property on="image::11" class="ImageControl"("Caption.Text"="GUIdevice 11") -> ()  [unwired: 2 in, 2 out]
      n169 = property on="image::12" class="ImageControl"("Caption.Text"="GUIdevice 12") -> ()  [unwired: 2 in, 2 out]
      n170 = Array To Cluster(array=w33) -> (cluster=→"Cameras":T7)
      n171 = property on="CCDs" class="Ring (strict)"("Strings []"=w33) -> ()  [unwired: 2 in, 2 out]
      n172 = Tick Count (ms)() -> (millisecond timer value=→"millisecond timer value":u32)
      n173 = property on="Feedback Global" class="Bool (strict)"("Value"=FALSE ("Feedback Global")) -> ()  [unwired: 2 in, 2 out]
      n174 = call "supergui create stop queue.vi"() -> ("STOP Queue out"=w35:refnum<queue>)  [unwired: 11 in]
      n175 = Create User Event(user event datatype=T5 {"EventEnum"=enum."new data", "Device name"="Device name"} ("New Event")) -> (user event=w193:refnum<user-event>, error out=w195:errorcluster)  [unwired: 1 in]
      "tcp data event" <- w193
      n176 = control-ref of="This Application"() -> (w194:refnum<vi>)
      n177 = control-ref of="This VI"() -> (w198:refnum<vi>)
      n178 = Current VI's Menubar() -> (w197:refnum<k9>)
      n179 = call "GUI_Master_subvi_reentrant_queues.vi"("STOP Queue in"=w35, "This Application"=w194, "error in (no error)"=w195, "tcp data event"=w193, "Caller menu reference"=w197, "Caller VI ref"=w198) -> ("error out"=→"error IO 2":errorcluster)  [unwired: 5 in]
      n180 = while {
        tunnel: w33 -> [w201]
        tunnel: [w201] -> w32
        stop <- "stop" stop-if-true
        n181 = Wait (ms)(milliseconds to wait=u32 500) -> ()  [unwired: 1 out]
      }
      n182 = for {
        tunnel: w32 -> [w205] mode=indexing
        tunnel: errorcluster {"status"=FALSE, "code"=0, "source"=""} ("error out") -> [w204]
        tunnel: [w203] -> w113
        n183 = call "IMAQ Dispose"("Image"=w205, "error in (no error)"=w204) -> ("error out"=w203:errorcluster)  [unwired: 4 in]
      }
      "error out 2" <- w113
    }
  }
